vi "DecodeButton.vi"(10 "Button":bool) -> (1 "False to True":bool, 3 "Button State":T1(ring))   [LabVIEW 2011]
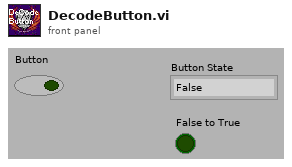
[diagram p1: front panel]
types:
  T1 = enum16{"False", "FalseToTrue", "True", "TrueToFalse"}
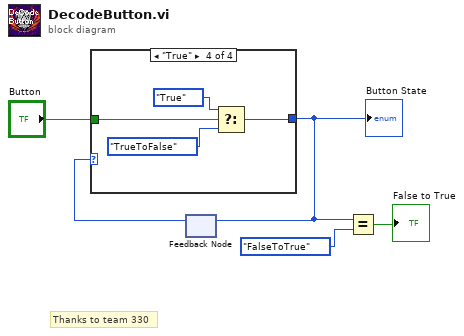
[diagram p0: block diagram]
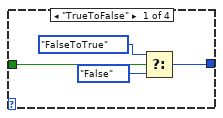
[diagram p2: hidden frame]
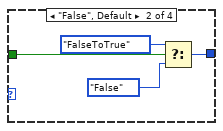
[diagram p3: hidden frame]
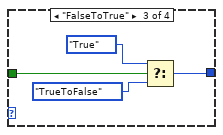
[diagram p4: hidden frame]
diagram:
  # "Thanks to team 330"
  n1 = feedback #1() -> (w1:T1)  [unwired: 1 out]
  n2 = case shown="\"True\"" w1 {
    tunnel: "Button" -> [w8 w13 w16 w19]
    tunnel: [w7 w10 w15 w18] -> w2
    frame "TrueToFalse" {
      n3 = Select(t=T1."FalseToTrue" ("y"), s=w8, f=T1."False") -> (s? t:f=w7:T1)
    }
    frame "False", Default {
      n4 = Select(t=T1."FalseToTrue", s=w13, f=T1."False" ("Button State")) -> (s? t:f=w10:T1)
    }
    frame "FalseToTrue" {
      n5 = Select(t=T1."True" ("y"), s=w16, f=T1."TrueToFalse") -> (s? t:f=w15:T1)
    }
    frame "True" {
      n6 = Select(t=T1."True" ("y"), s=w19, f=T1."TrueToFalse") -> (s? t:f=w18:T1)
    }
  }
  "Button State" <- w2
  n7 = feedback-in #1(w2) -> ()
  n8 = Equal?(x=w2, y=T1."FalseToTrue") -> (x = y?=→"False to True":bool)
